vi "Create Data File.vi"(8 "Error IN":errorcluster, 10 "Trial#":i16, 11 "Save Directory IN":path) -> (0 "Error OUT":errorcluster, 3 "Data File Path OUT":path)   [LabVIEW 2018]
panel:
  # "INPUTS"
  # "OUTPUTS"
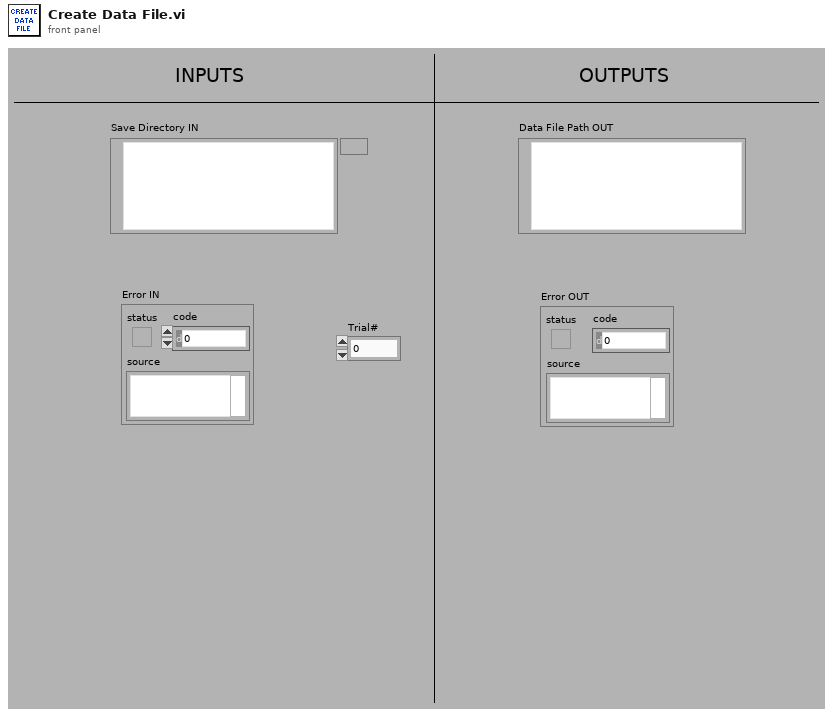
[diagram p1: front panel]
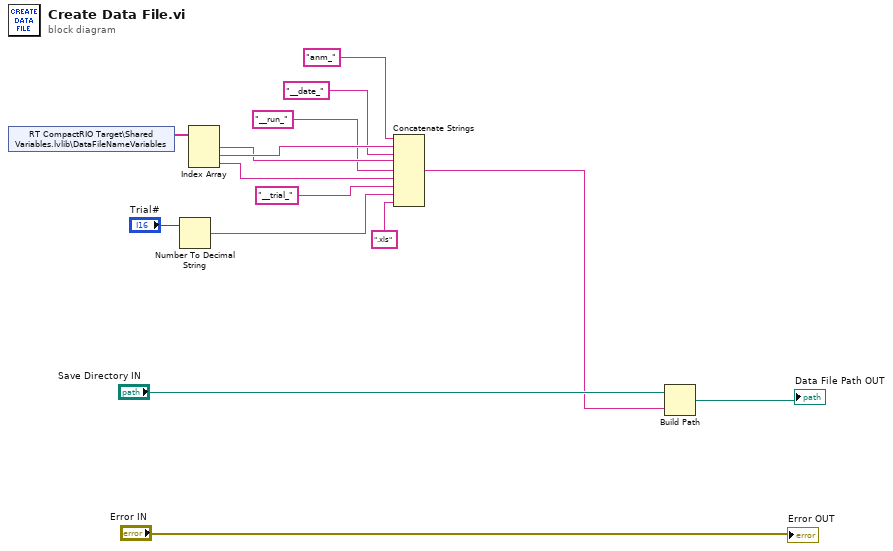
[diagram p0: block diagram]
diagram:
  n1 = shared-variable "RT CompactRIO Target\\Shared Variables.lvlib\\DataFileNameVariables"() -> (w12:string[])  [unwired: 1 in, 1 out]
  n2 = Number To Decimal String(number="Trial#") -> (decimal integer string=w4:string)  [unwired: 1 in]
  n3 = Index Array(array=w12) -> (element #1=w8:string, element #2=w10:string, element #3=w6:string)  [unwired: 3 in]
  n4 = Concatenate Strings("anm_", w10, "__date_", w8, "__run_", w6, "__trial_", w4, ".xls") -> (w2:string)
  n5 = Build Path(base path="Save Directory IN", name or relative path=w2) -> (appended path=→"Data File Path OUT":path)
  "Error OUT" <- "Error IN"
